vi "DO N Samples（Host）.vi"() -> ()   [LabVIEW 2019]
uses:
  <vilib>/FPGAPlugInAG/ELVIS III/niLvFpga_Open_ELVIS III.vi
  <vilib>/rvi/interface/common/dynamic/niFpgaDynamicAddResources.vi
  <vilib>/rvi/interface/common/niFpgaWaitOnOcc.vi
  <vilib>/Utility/error.llb/Error Cluster From Error Code.vi
  <vilib>/FPGAPlugInAG/Dynamic/niLvFpga_Run_Dynamic.vi
  <vilib>/rvi/errors/niLvFpgaAdjustHostInterfaceError.vi
  <vilib>/FPGAPlugInAG/Dynamic/niLvFpga_Close_Dynamic.vi
  <vilib>/rvi/interface/nirviOpenFPGA/nirviOpenFPGA.xnode
  FPGA Bitfiles/digitalio-fpga_FPGATarget_DONSamples_Y7cbZnkCE40.lvbitx
  DO N Samples.vi
  <vilib>/rvi/interface/nirviMethod/nirviMethod.xnode
  <vilib>/rvi/interface/nirviReadWriteControl/nirviReadWriteControl.xnode
  <vilib>/rvi/interface/nirviCloseFPGA/nirviCloseFPGA.xnode
  <vilib>/FPGAPlugInAG/Dynamic/niLvFpga_ConfigureFifo_Dynamic.vi
  <vilib>/rvi/errors/niLvFpgaMergeErrorWithErrorCode.vi
  NiFpgaLv.dll
  <vilib>/rvi/interface/Simulation/niFpgaSimulationCallBeginRW.vi
  <vilib>/FPGAPlugInAG/Dynamic/niLvFpga_WriteFifo_Dynamic.vi
  <vilib>/FPGAPlugInAG/Dynamic/niLvFpga_StopFifo_Dynamic.vi
panel:
  out "B":digitalwaveform(graph)
  out "A":digitalwaveform(graph)
  in  "DO.B.DMA_ENA":bool[](array[boolean])=[FALSE, FALSE, FALSE, FALSE, FALSE, FALSE, FALSE, FALSE, FALSE, FALSE, FALSE, FALSE, FALSE, FALSE, FALSE, FALSE, FALSE, FALSE, FALSE, FALSE]
  in  "DO.A.DMA_ENA":bool[](array[boolean])=[FALSE, FALSE, FALSE, FALSE, FALSE, FALSE, FALSE, FALSE, FALSE, FALSE, FALSE, FALSE, FALSE, FALSE, FALSE, FALSE, FALSE, FALSE, FALSE, FALSE]
  in  "停止":bool
  in  "DO.B.DMA_CNTR":u16=1000
  in  "DO.A.DMA_CNTR":u16=1000
  in  "B.DIR":bool[](array[boolean])=[FALSE, FALSE, FALSE, FALSE, FALSE, FALSE, FALSE, FALSE, FALSE, FALSE, FALSE, FALSE, FALSE, FALSE, FALSE, FALSE, FALSE, FALSE, FALSE, FALSE]
  in  "A.DIR":bool[](array[boolean])=[FALSE, FALSE, FALSE, FALSE, FALSE, FALSE, FALSE, FALSE, FALSE, FALSE, FALSE, FALSE, FALSE, FALSE, FALSE, FALSE, FALSE, FALSE, FALSE, FALSE]
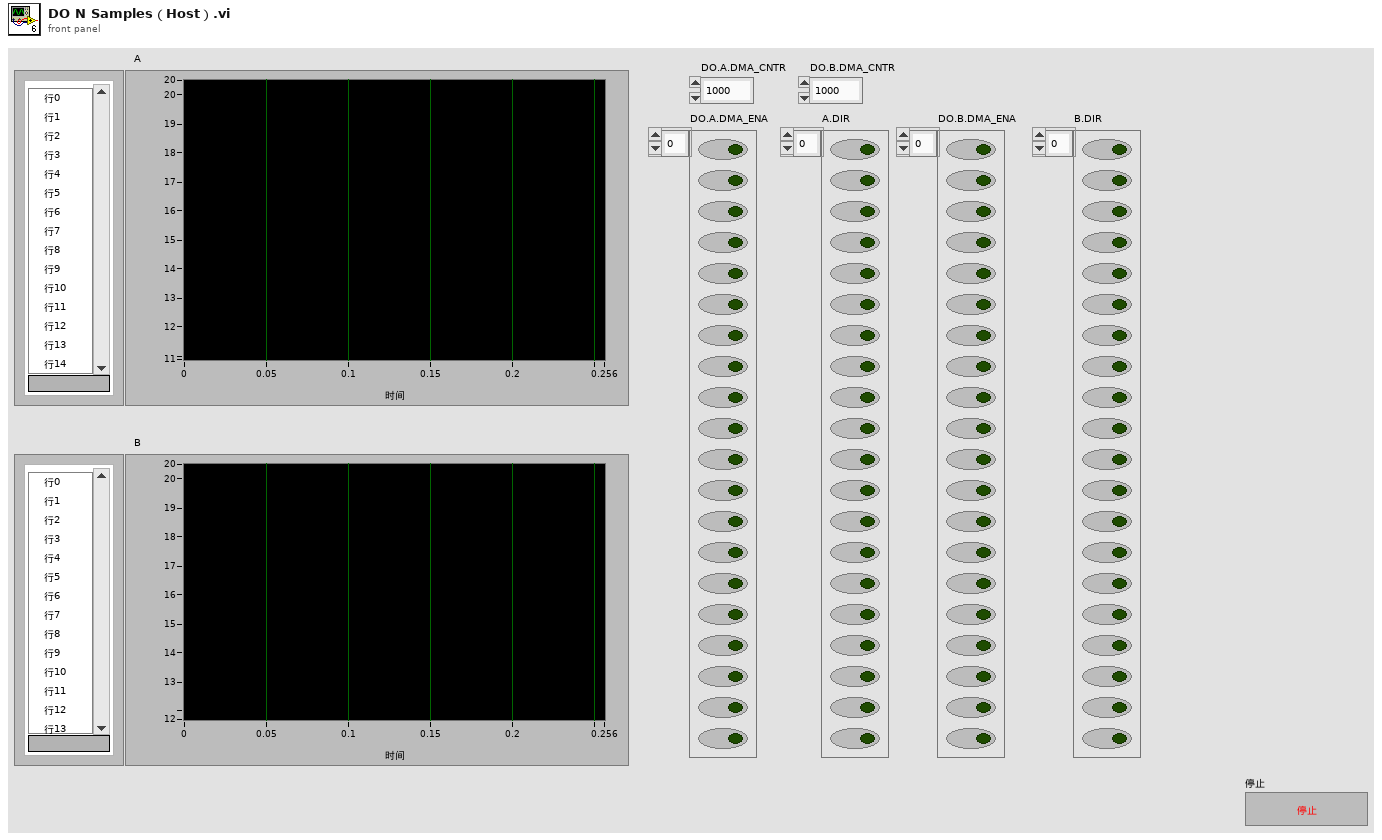
[diagram p1: front panel]
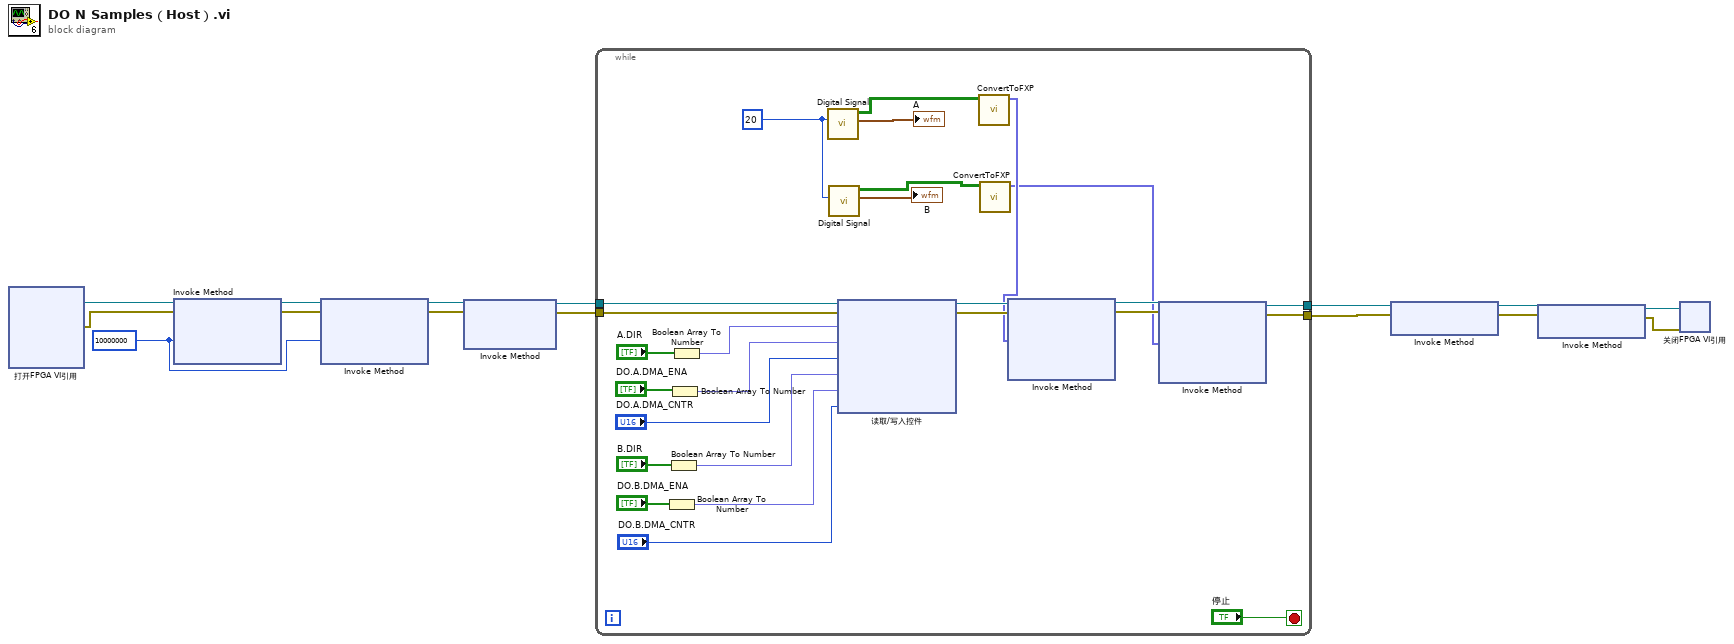
[diagram p0: block diagram]
diagram:
  w11 = u32 10000000 ("请求的深度")
  n1 = xnode "打开FPGA VI引用"() -> ("FPGA VI引用输出"=w15:refnum<k20>, "错误输出"=w12:errorcluster)  [unwired: 2 in]
  n2 = xnode "Invoke Method"("FPGA VI引用输入"=w15, "错误输入"=w12, "请求的深度"=w11) -> ("FPGA VI引用输出"=w13:refnum<k20>, "错误输出"=w14:errorcluster)  [unwired: 1 out]
  n3 = xnode "Invoke Method"("FPGA VI引用输入"=w13, "错误输入"=w14, "请求的深度"=w11) -> ("FPGA VI引用输出"=w9:refnum<k20>, "错误输出"=w10:errorcluster)  [unwired: 1 out]
  n4 = xnode "Invoke Method"("FPGA VI引用输入"=w9, "错误输入"=w10) -> ("FPGA VI引用输出"=w8:refnum<k20>, "错误输出"=w7:errorcluster)  [unwired: 1 in]
  n5 = while {
    tunnel: w8 -> [w40]
    tunnel: w7 -> [w41]
    tunnel: [w18] -> w6
    tunnel: [w17] -> w5
    stop <- "停止" stop-if-true
    w27 = u32 20 ("number of signals")
    n6 = Boolean Array To Number ("布尔数组至数值转换")(Boolean array="DO.B.DMA_ENA") -> (number=w31:fxp<+,20,20>)
    n7 = Boolean Array To Number ("布尔数组至数值转换")(Boolean array="B.DIR") -> (number=w32:fxp<+,20,20>)
    n8 = Boolean Array To Number ("布尔数组至数值转换")(Boolean array="DO.A.DMA_ENA") -> (number=w34:fxp<+,20,20>)
    n9 = Boolean Array To Number ("布尔数组至数值转换")(Boolean array="A.DIR") -> (number=w35:fxp<+,20,20>)
    n10 = call "Digital Signal.vi"("number of signals"=w27) -> ("digital waveform"=→"A":digitalwaveform, "数组"=w23:bool[][])  [unwired: 8 in, 1 out]
    n11 = call "Digital Signal.vi"("number of signals"=w27) -> ("digital waveform"=→"B":digitalwaveform, "数组"=w24:bool[][])  [unwired: 8 in, 1 out]
    n12 = xnode "读取/写入控件"("FPGA VI引用输入"=w40, "错误输入"=w41, "DIO.A_19:0.DIR"=w35, "DO.A.DMA_ENA"=w34, "DO.A.DMA_CNTR"="DO.A.DMA_CNTR", "DIO.B_19:0.DIR"=w32, "DO.B.DMA_ENA"=w31, "DO.B.DMA_CNTR"="DO.B.DMA_CNTR") -> ("FPGA VI引用输出"=w28:refnum<k20>, "错误输出"=w29:errorcluster)
    n13 = call "ConvertToFXP.vi"("Digtal"=w23) -> ("FXP"=w20:fxp<+,20,20>[])  [unwired: 10 in]
    n14 = call "ConvertToFXP.vi"("Digtal"=w24) -> ("FXP"=w19:fxp<+,20,20>[])  [unwired: 10 in]
    n15 = xnode "Invoke Method"("FPGA VI引用输入"=w28, "错误输入"=w29, "数据"=w20) -> ("FPGA VI引用输出"=w21:refnum<k20>, "错误输出"=w22:errorcluster)  [unwired: 1 in, 1 out]
    n16 = xnode "Invoke Method"("FPGA VI引用输入"=w21, "错误输入"=w22, "数据"=w19) -> ("FPGA VI引用输出"=w17:refnum<k20>, "错误输出"=w18:errorcluster)  [unwired: 1 in, 1 out]
  }
  n17 = xnode "Invoke Method"("FPGA VI引用输入"=w5, "错误输入"=w6) -> ("FPGA VI引用输出"=w3:refnum<k20>, "错误输出"=w4:errorcluster)
  n18 = xnode "Invoke Method"("FPGA VI引用输入"=w3, "错误输入"=w4) -> ("FPGA VI引用输出"=w1:refnum<k20>, "错误输出"=w2:errorcluster)
  n19 = xnode "关闭FPGA VI引用"("FPGA VI引用输入"=w1, "错误输入"=w2) -> ()  [unwired: 1 out]
